vi "Update.vi"(8 "error in (no error)":errorcluster, 11 "Deck in":refnum<class "Deck.lvclass">) -> (0 "error out":errorcluster, 2 "Audio Block":dbl[][](array[numeric]), 3 "Deck out":refnum<class "Deck.lvclass">)   [LabVIEW 2019, in "Deck.lvclass"]
uses:
  Deck.lvclass
  Deck.lvclass/Deck.ctl
  State.ctl
  Libraries/Audio Processing/Adjust Sample Size.vi
  Libraries/Globals/Constants.vi
  <vilib>/gmath/NI_Gmath.lvlib
  Libraries/User Interface/User Interface.lvlib
  Libraries/Audio Processing/Audio Processing.lvlib
  Libraries/Messaging/Messaging.lvlib
  Libraries/Globals/Globals.lvlib
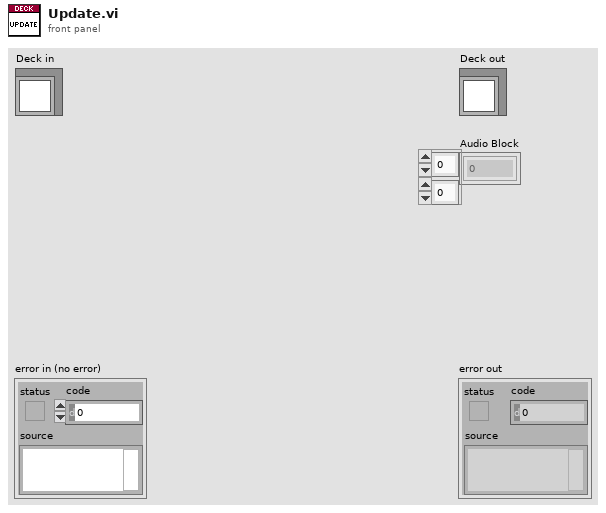
[diagram p1: front panel]
types:
  T1 = typedef "Deck.lvclass/State.ctl" = enum16{"No Track", "Loading", "Active", "Scratching", "Brake", "Backspin"}
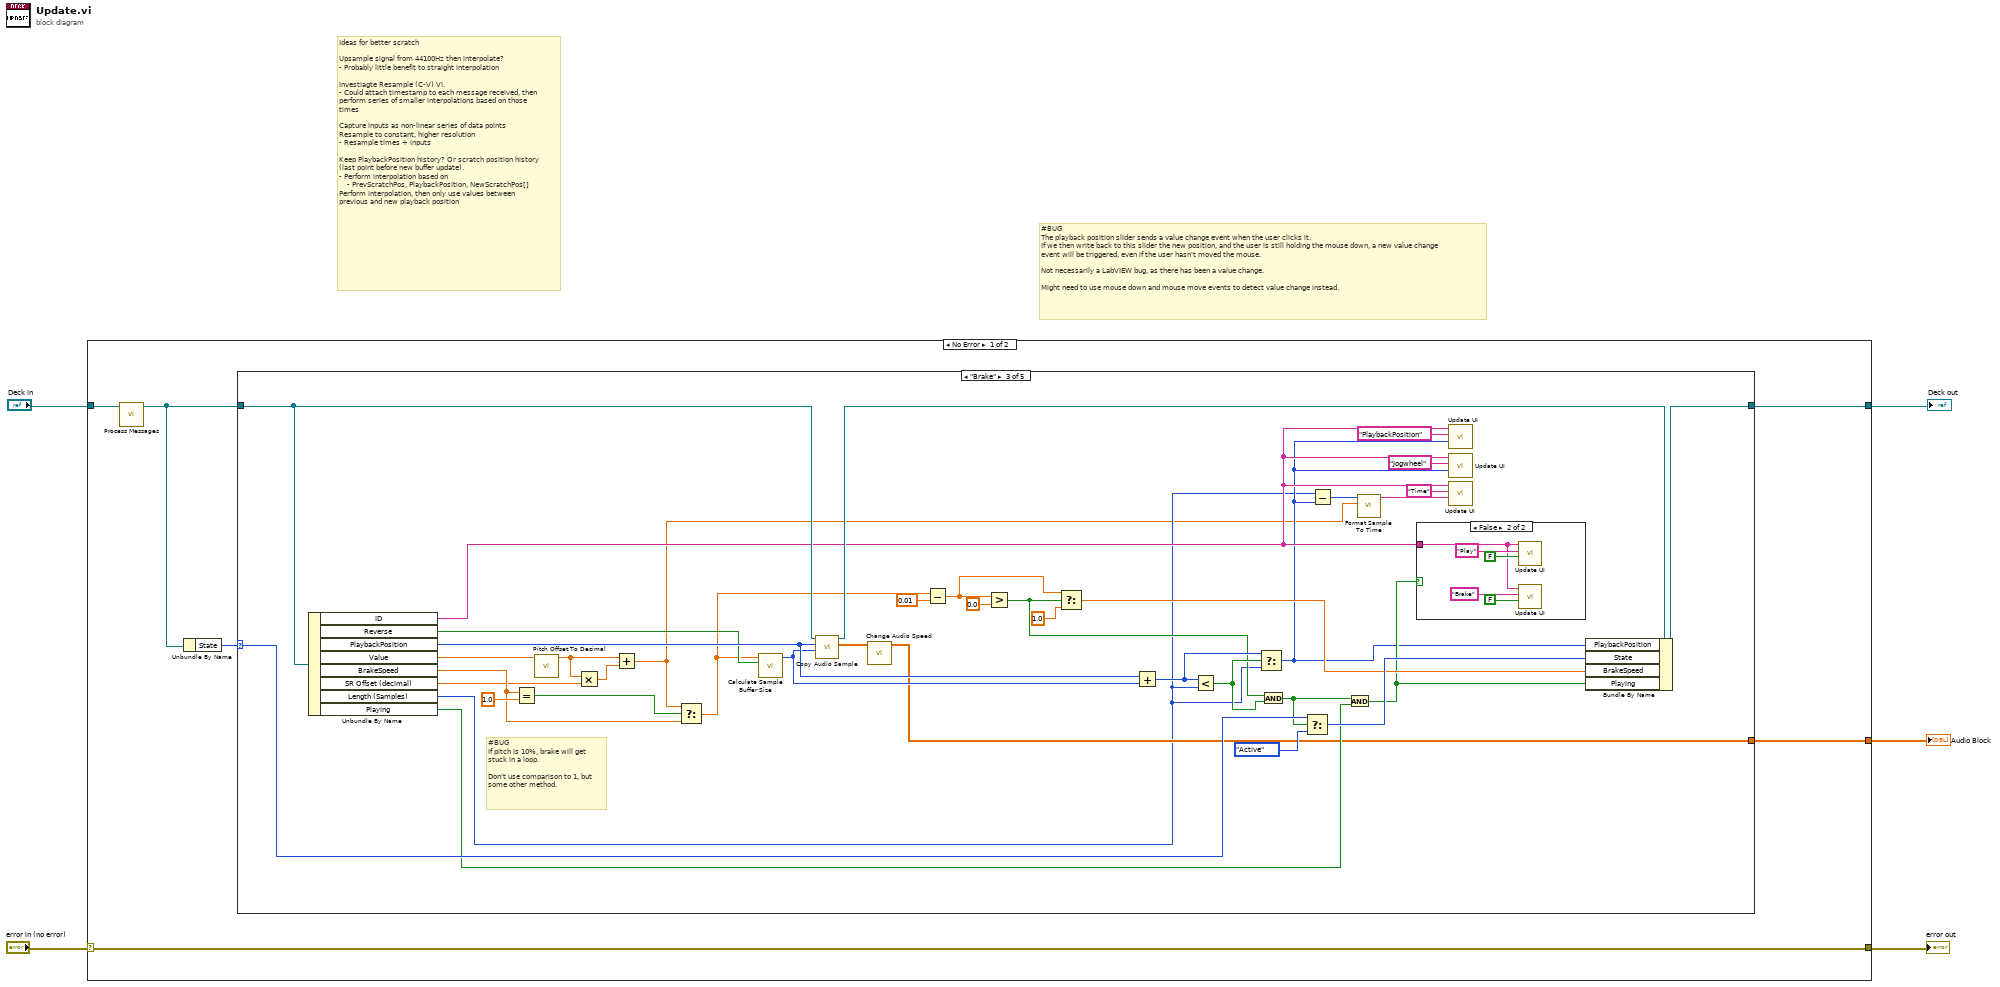
[diagram p0: block diagram]
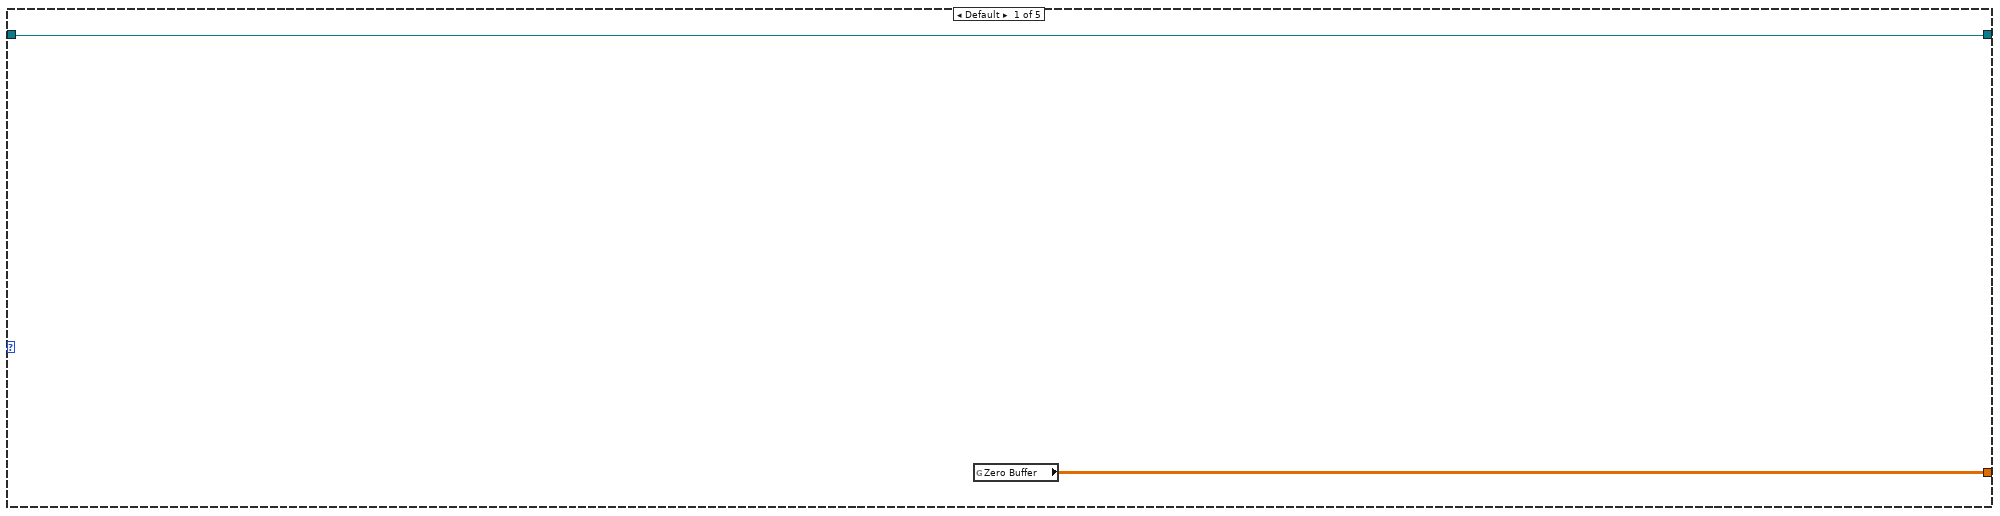
[diagram p2: hidden frame]
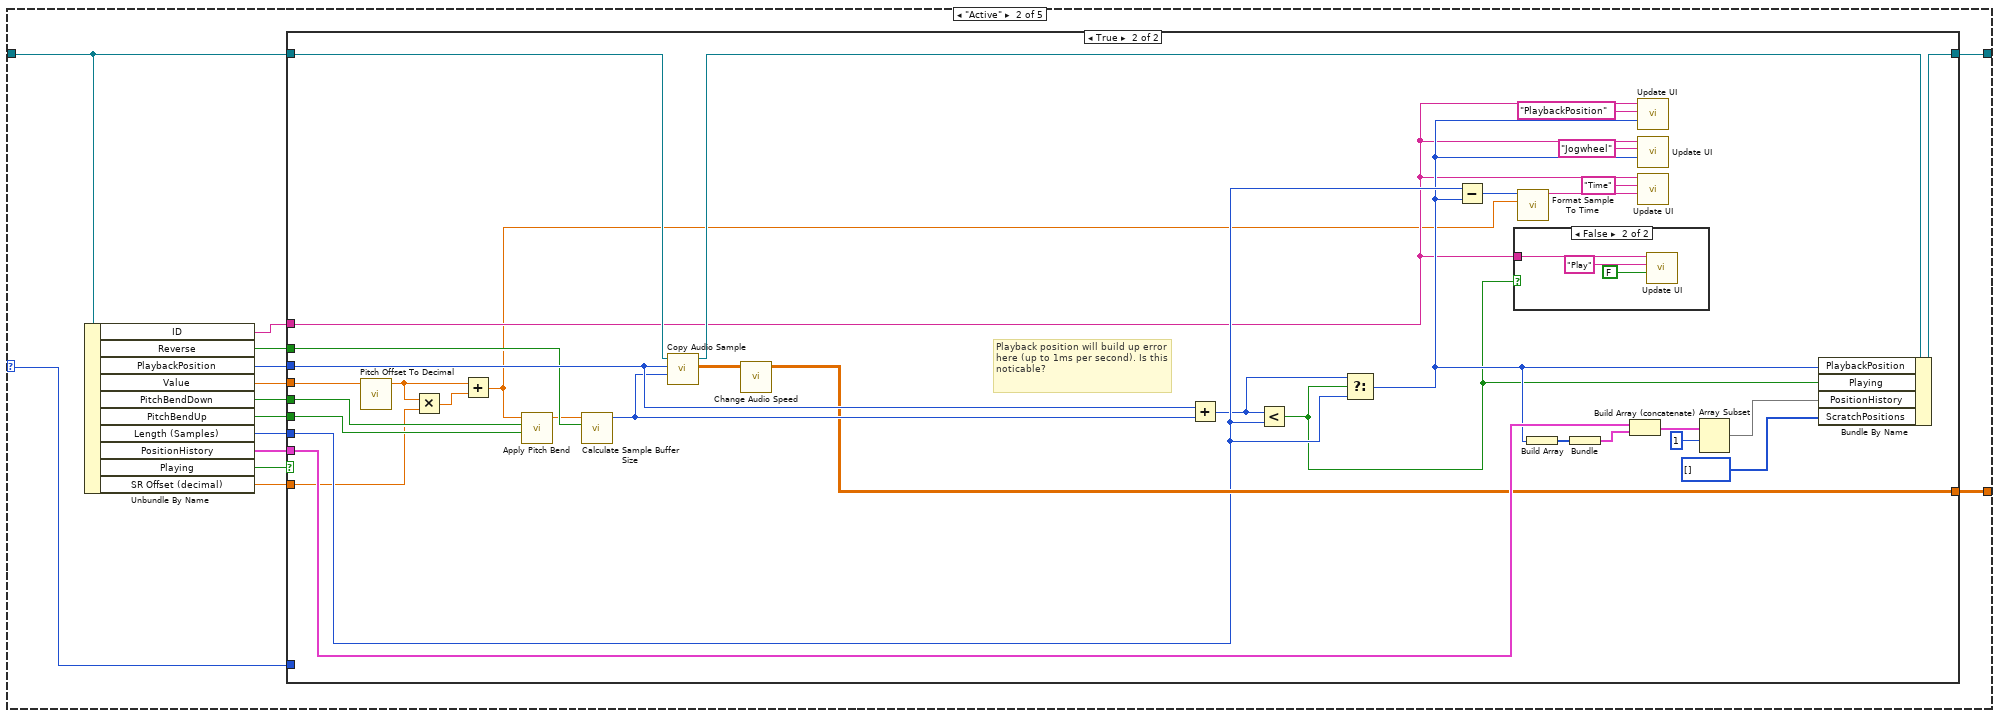
[diagram p3: hidden frame]
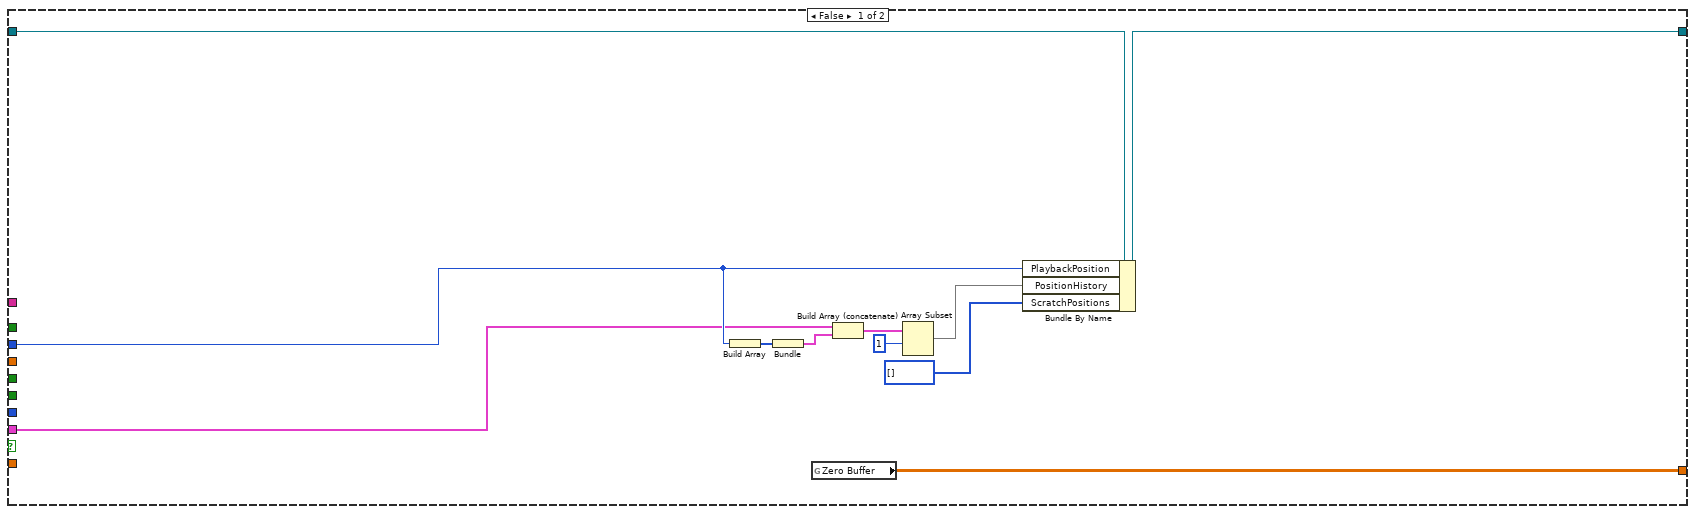
[diagram p4: hidden frame]
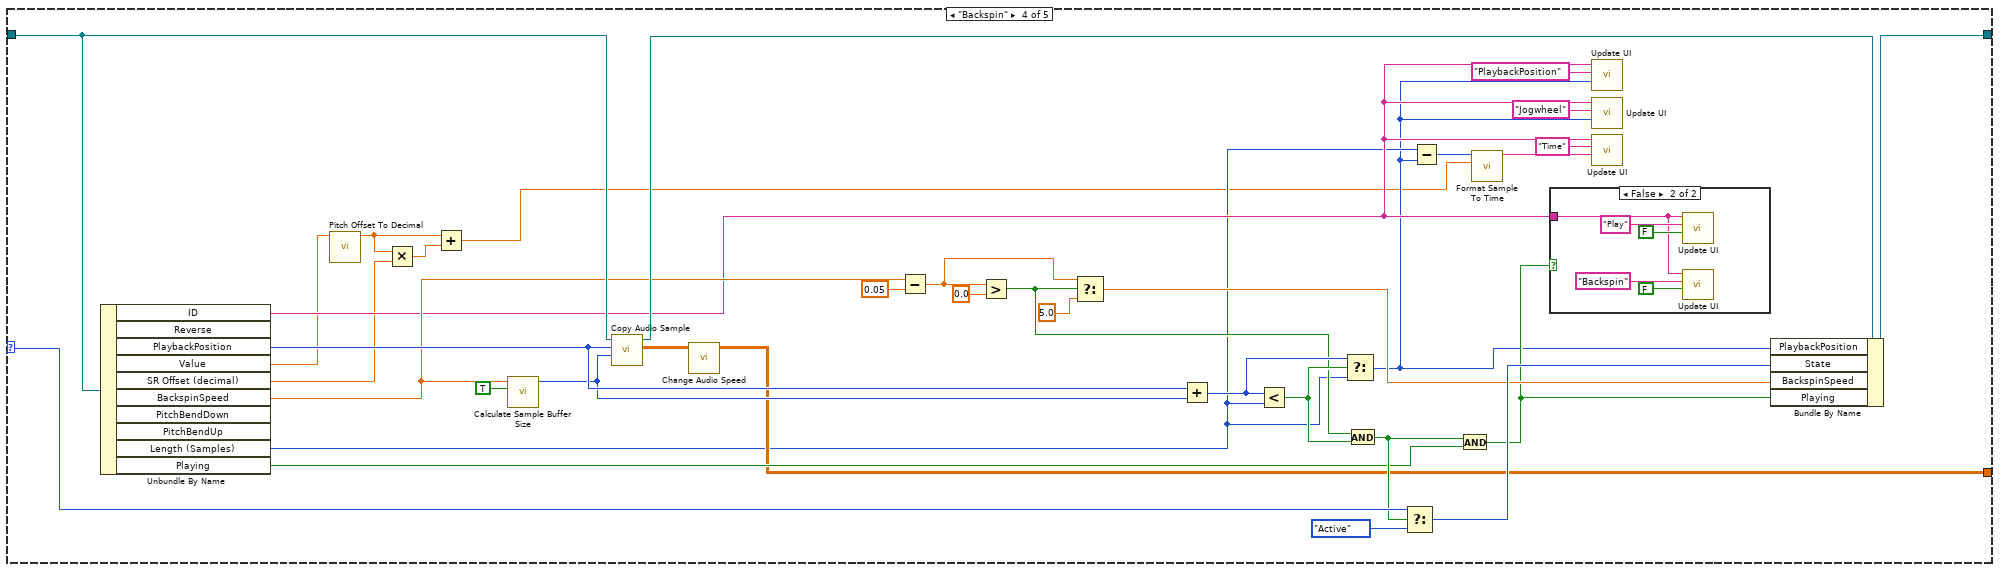
[diagram p7: hidden frame]
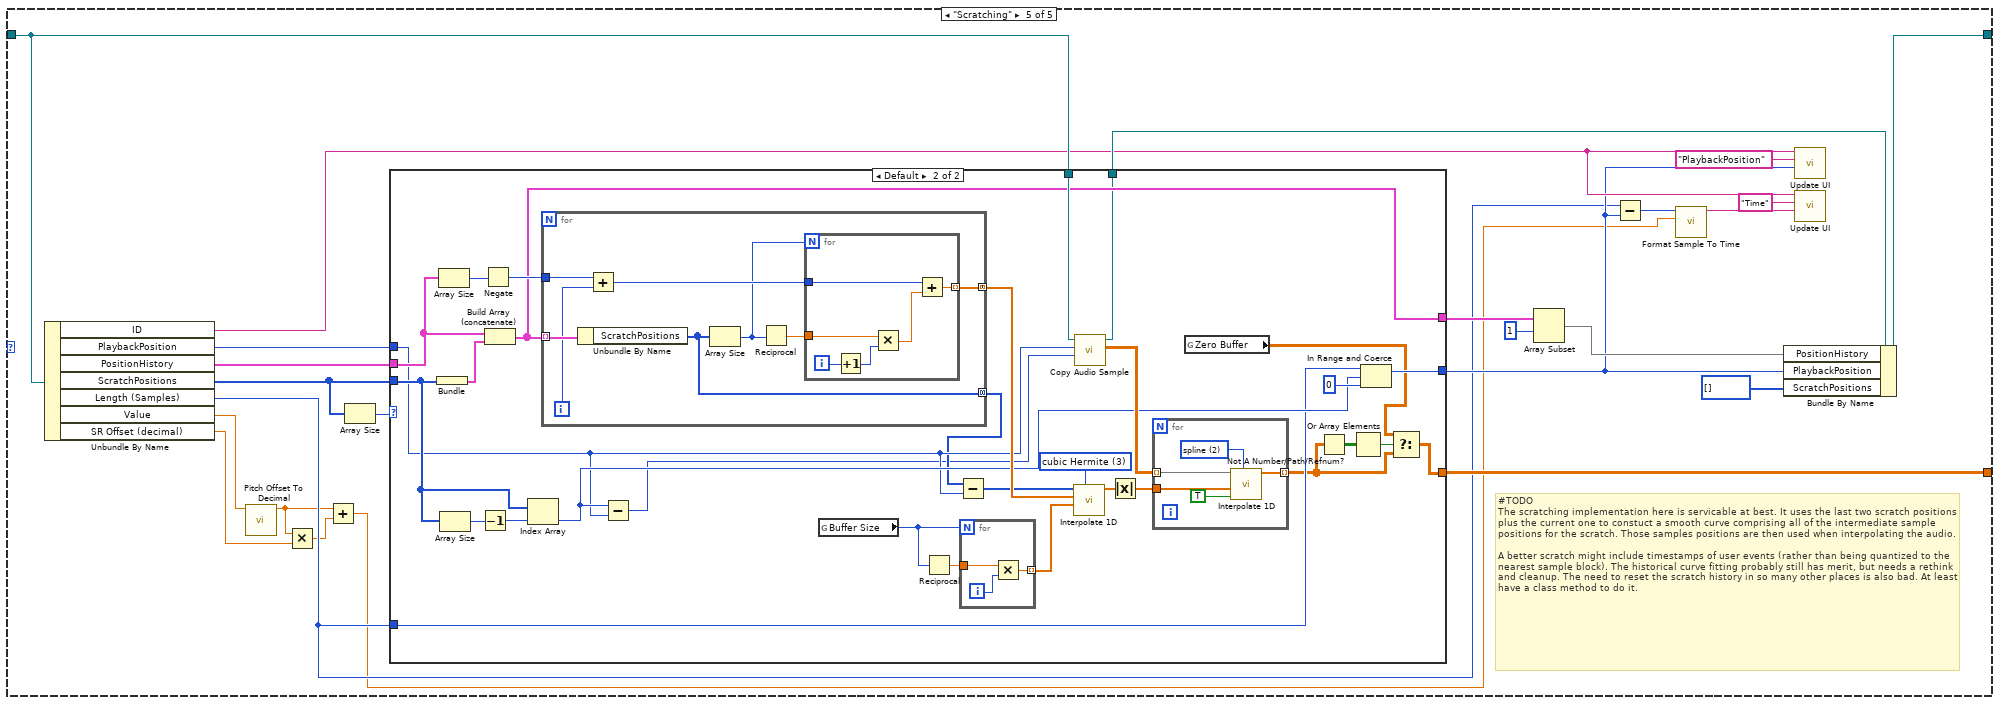
[diagram p9: hidden frame]
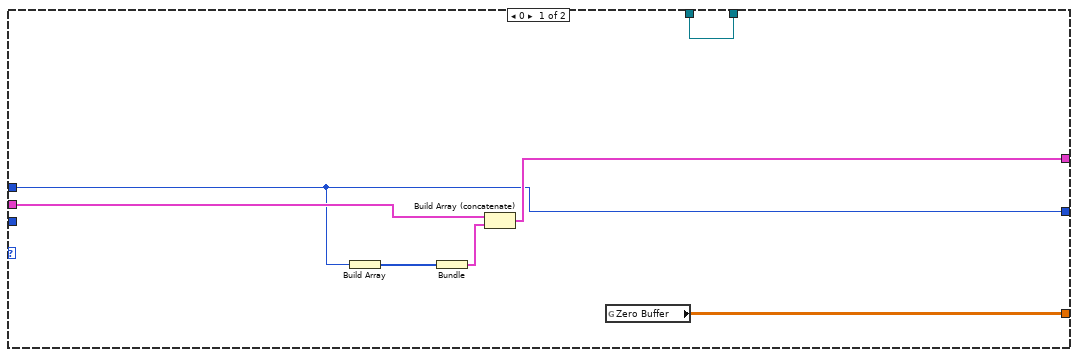
[diagram p10: hidden frame]
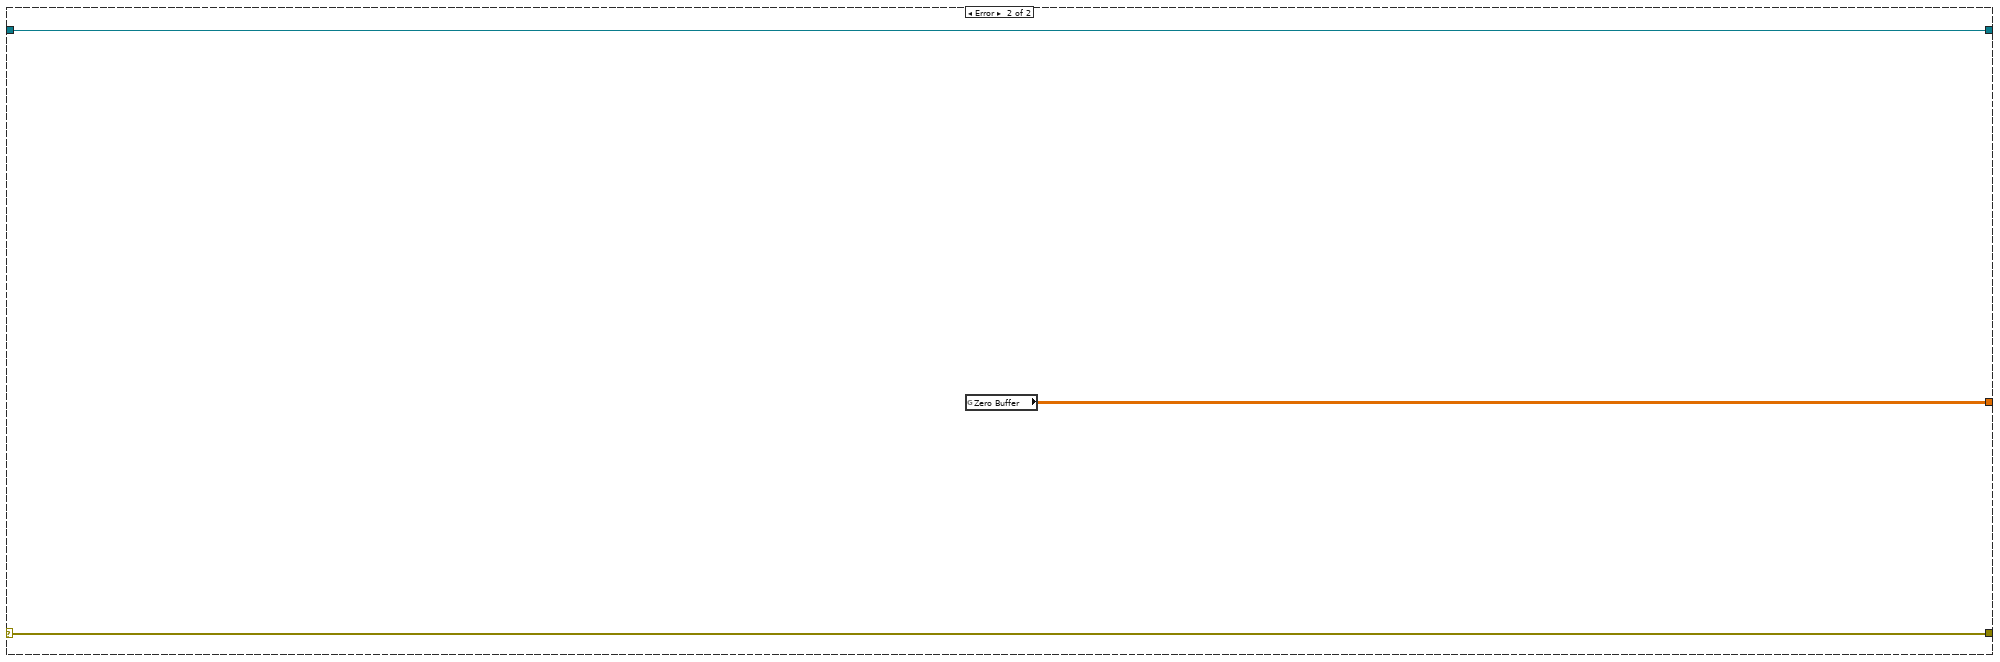
[diagram p11: hidden frame]
diagram:
  # "Ideas for better scratch\n\nUpsample signal from 44100Hz then interpolate?\n- Probably little benefit to straight interpolation\n\nInvestiagte Resample (C-V) VI.\n- Could attach timestamp to each message received, then perform series of smaller interpolations based on those times\n\nCapture inputs as non-linear series of data points\nResample to constant, higher resolution\n- Resample times + inputs\n\nKeep PlaybackPosition history? Or scratch position history (last point before new buffer update).\n- Perform interpolation based on\n    - PrevScratchPos, PlaybackPosition, NewScratchPos[]\nPerform interpolation, then only use values between previous and new playback position"
  # "#BUG\nThe playback position slider sends a value change event when the user clicks it.\nIf we then write back to this slider the new position, and the user is still holding the mouse down, a new value change event will be triggered, even if the user hasn't moved the mouse.\n\nNot necessarily a LabVIEW bug, as there has been a value change.\n\nMight need to use mouse down and mouse move events to detect value change instead."
  n1 = case shown="No Error" "error in (no error)" {
    selector: "error in (no error)" -> [w11 w246]
    tunnel: [w11 w246] -> w4
    tunnel: [w9 w245] -> w2
    tunnel: "Deck in" -> [w6 w245]
    tunnel: [w8 w244] -> w1
    frame No Error {
      n2 = call "Process Messages.vi"("Deck in"=w6) -> ("Deck out"=w7:refnum<class "Deck.lvclass">)  [unwired: 9 in, 1 out]
      n3 = Unbundle By Name(w7) -> ("State"=w10:T1)
      n4 = case shown="\"Brake\"" w10 {
        selector: w10 -> [_ w20 w108 w149 _]
        tunnel: [w13 w27 w113 w154 w183] -> w9
        tunnel: w7 -> [w13 w26 w111 w152 w181]
        tunnel: [w12 w24 w87 w133 w172] -> w8
        frame Default {
          n5 = global read "Constants.vi" "Zero Buffer"() -> (w12:dbl[][])
        }
        frame "Active" {
          n6 = Unbundle By Name(w26) -> ("ID"=w16:string, "Reverse"=w15:bool, "PlaybackPosition"=w25:i32, "Value"=w22:dbl, "PitchBendDown"=w23:bool, "PitchBendUp"=w21:bool, "Length (Samples)"=w18:i32, "PositionHistory"=w19:cluster{"Positions":i32[]}[], "Playing"=w17:bool, "SR Offset (decimal)"=w14:dbl)
          n7 = case shown="True" w17 {
            tunnel: [w31 w71] -> w27
            tunnel: w26 -> [w30 w69]
            tunnel: w25 -> [w29 w68]
            tunnel: [w38 w56] -> w24
            tunnel: w23 -> [_ w42]
            tunnel: w22 -> [_ w60]
            tunnel: w21 -> [_ w43]
            tunnel: w20 -> [_ _]
            tunnel: w19 -> [w28 w65]
            tunnel: w16 -> [_ w46]
            tunnel: w18 -> [_ w55]
            tunnel: w15 -> [_ w59]
            tunnel: w14 -> [_ w41]
            frame False {
              n8 = Build Array(w29) -> (w34:i32[])
              n9 = Bundle(w34) -> (w33:cluster{i32[]})  [unwired: 1 in]
              n10 = global read "Constants.vi" "Zero Buffer"() -> (w38:dbl[][])
              n11 = Build Array (concatenate)(w28, w33) -> (w37:cluster{"Positions":i32[]}[])
              n12 = Array Subset(array=w37, index=1) -> (w35:cluster{"Positions":i32[]}[])  [unwired: 1 in]
              n13 = Bundle By Name(cluster=w30, "PlaybackPosition"=w29, "PositionHistory"=w35, "ScratchPositions"=i32[] []) -> (w31:refnum<class "Deck.lvclass">)
            }
            frame True {
              # "Playback position will build up error here (up to 1ms per second). Is this noticable?"
              n14 = call "Pitch Offset To Decimal.vi"("Pitch Offset (%)"=w60) -> ("Pitch (decimal)"=w40:dbl)  [unwired: 10 in]
              n15 = Multiply(x=w40, y=w41) -> (x*y=w39:dbl)
              n16 = Add(x=w40, y=w39) -> (x+y=w45:dbl)
              n17 = call "Apply Pitch Bend.vi"("Pitch Bend Up (F)"=w43, "Pitch Bend Down (F)"=w42, "Pitch (decimal) In"=w45) -> ("Pitch (decimal) Out"=w44:dbl)  [unwired: 8 in]
              n18 = call "Calculate Sample Buffer Size.vi"("Reverse (F)"=w59, "Speed Multiplier"=w44) -> ("Sample Size"=w58:i32)  [unwired: 9 in]
              n19 = call "Copy Audio Sample.vi"("Length"=w58, "Offset"=w68, "Deck in"=w69) -> ("Audio Block"=w57:dbl[][], "Deck out"=w70:refnum<class "Deck.lvclass">)  [unwired: 6 in, 1 out]
              n20 = call "Change Audio Speed.vi"("Audio Block"=w57) -> ("Interpolated Audio"=w56:dbl[][])  [unwired: 10 in]
              n21 = Add(x=w68, y=w58) -> (x+y=w54:i32)
              n22 = Less?(x=w54, y=w55) -> (x < y?=w47:bool)
              n23 = Select(t=w54, s=w47, f=w55) -> (s? t:f=w50:i32)
              n24 = Subtract(x=w55, y=w50) -> (x-y=w53:i32)
              n25 = case shown="False" w47 {
                tunnel: w46 -> [_ w72]
                frame True {
                }
                frame False {
                  n26 = call "Update UI.vi"("Data"=FALSE, "Target"="Play" ("format string"), "ID"=w72) -> ()  [unwired: 8 in, 1 out]
                }
              }
              n27 = call "Format Sample To Time.vi"("Pitch (decimal) (1)"=w45, "Samples"=w53) -> ("Formatted Time"=w49:string)  [unwired: 9 in]
              n28 = Build Array(w50) -> (w63:i32[])
              n29 = Bundle(w63) -> (w62:cluster{i32[]})  [unwired: 1 in]
              n30 = Build Array (concatenate)(w65, w62) -> (w67:cluster{"Positions":i32[]}[])
              n31 = call "Update UI.vi"("Data"=w50, "Target"="PlaybackPosition" ("format string"), "ID"=w46) -> ()  [unwired: 8 in, 1 out]
              n32 = call "Update UI.vi"("Data"=w50, "Target"="Jogwheel" ("format string"), "ID"=w46) -> ()  [unwired: 8 in, 1 out]
              n33 = call "Update UI.vi"("Data"=w49, "Target"="Time" ("format string"), "ID"=w46) -> ()  [unwired: 8 in, 1 out]
              n34 = Array Subset(array=w67, index=1) -> (w64:cluster{"Positions":i32[]}[])  [unwired: 1 in]
              n35 = Bundle By Name(cluster=w70, "PlaybackPosition"=w50, "Playing"=w47, "PositionHistory"=w64, "ScratchPositions"=i32[] []) -> (w71:refnum<class "Deck.lvclass">)
            }
          }
        }
        frame "Brake" {
          # "#BUG\nIf pitch is 10%, brake will get stuck in a loop.\n\nDon't use comparison to 1, but some other method."
          n36 = Unbundle By Name(w111) -> ("ID"=w81:string, "Reverse"=w90:bool, "PlaybackPosition"=w110:i32, "Value"=w92:dbl, "BrakeSpeed"=w96:dbl, "SR Offset (decimal)"=w76:dbl, "Length (Samples)"=w79:i32, "Playing"=w94:bool)
          n37 = Equal?(x=w96, y=1.0) -> (x = y?=w97:bool)
          n38 = call "Pitch Offset To Decimal.vi"("Pitch Offset (%)"=w92) -> ("Pitch (decimal)"=w77:dbl)  [unwired: 10 in]
          n39 = Multiply(x=w77, y=w76) -> (x*y=w78:dbl)
          n40 = Add(x=w77, y=w78) -> (x+y=w75:dbl)
          n41 = Select(t=w75, s=w97, f=w96) -> (s? t:f=w89:dbl)
          n42 = call "Calculate Sample Buffer Size.vi"("Reverse (F)"=w90, "Speed Multiplier"=w89) -> ("Sample Size"=w88:i32)  [unwired: 9 in]
          n43 = call "Copy Audio Sample.vi"("Length"=w88, "Offset"=w110, "Deck in"=w111) -> ("Audio Block"=w91:dbl[][], "Deck out"=w112:refnum<class "Deck.lvclass">)  [unwired: 6 in, 1 out]
          n44 = call "Change Audio Speed.vi"("Audio Block"=w91) -> ("Interpolated Audio"=w87:dbl[][])  [unwired: 10 in]
          n45 = Subtract(x=w89, y=0.01) -> (x-y=w99:dbl)
          n46 = Greater?(x=w99, y=0.0) -> (0:w102:bool)
          n47 = Select(t=w99, s=w102, f=1.0 ("t")) -> (s? t:f=w101:dbl)
          n48 = Add(x=w110, y=w88) -> (x+y=w109:i32)
          n49 = Less?(x=w109, y=w79) -> (x < y?=w103:bool)
          n50 = Select(t=w109, s=w103, f=w79) -> (s? t:f=w80:i32)
          n51 = And(x=w102, y=w103) -> (x .and. y?=w95:bool)
          n52 = Select(t=w108, s=w95, f=State."Active") -> (s? t:f=w107:T1)
          n53 = Subtract(x=w79, y=w80) -> (x-y=w86:i32)
          n54 = And(x=w95, y=w94) -> (x .and. y?=w93:bool)
          n55 = call "Format Sample To Time.vi"("Pitch (decimal) (1)"=w75, "Samples"=w86) -> ("Formatted Time"=w83:string)  [unwired: 9 in]
          n56 = case shown="False" w93 {
            tunnel: w81 -> [_ w114]
            frame True {
            }
            frame False {
              n57 = call "Update UI.vi"("Data"=FALSE, "Target"="Play" ("format string"), "ID"=w114) -> ()  [unwired: 8 in, 1 out]
              n58 = call "Update UI.vi"("Data"=FALSE, "Target"="Brake" ("format string"), "ID"=w114) -> ()  [unwired: 8 in, 1 out]
            }
          }
          n59 = call "Update UI.vi"("Data"=w80, "Target"="PlaybackPosition" ("format string"), "ID"=w81) -> ()  [unwired: 8 in, 1 out]
          n60 = call "Update UI.vi"("Data"=w80, "Target"="Jogwheel" ("format string"), "ID"=w81) -> ()  [unwired: 8 in, 1 out]
          n61 = call "Update UI.vi"("Data"=w83, "Target"="Time" ("format string"), "ID"=w81) -> ()  [unwired: 8 in, 1 out]
          n62 = Bundle By Name(cluster=w112, "PlaybackPosition"=w80, "State"=w107, "BrakeSpeed"=w101, "Playing"=w93) -> (w113:refnum<class "Deck.lvclass">)
        }
        frame "Backspin" {
          n63 = Unbundle By Name(w152) -> ("ID"=w127:string, "PlaybackPosition"=w151:i32, "Value"=w123:dbl, "SR Offset (decimal)"=w121:dbl, "BackspinSpeed"=w137:dbl, "Length (Samples)"=w125:i32, "Playing"=w138:bool)  [unwired: 3 out]
          n64 = call "Pitch Offset To Decimal.vi"("Pitch Offset (%)"=w123) -> ("Pitch (decimal)"=w119:dbl)  [unwired: 10 in]
          n65 = Multiply(x=w119, y=w121) -> (x*y=w122:dbl)
          n66 = Add(x=w119, y=w122) -> (x+y=w120:dbl)
          n67 = call "Calculate Sample Buffer Size.vi"("Reverse (F)"=TRUE, "Speed Multiplier"=w137) -> ("Sample Size"=w135:i32)  [unwired: 9 in]
          n68 = call "Copy Audio Sample.vi"("Length"=w135, "Offset"=w151, "Deck in"=w152) -> ("Audio Block"=w134:dbl[][], "Deck out"=w153:refnum<class "Deck.lvclass">)  [unwired: 6 in, 1 out]
          n69 = call "Change Audio Speed.vi"("Audio Block"=w134) -> ("Interpolated Audio"=w133:dbl[][])  [unwired: 10 in]
          n70 = Subtract(x=w137, y=0.05) -> (x-y=w140:dbl)
          n71 = Greater?(x=w140, y=0.0) -> (0:w143:bool)
          n72 = Select(t=w140, s=w143, f=5.0 ("t")) -> (s? t:f=w142:dbl)
          n73 = Add(x=w151, y=w135) -> (x+y=w150:i32)
          n74 = Less?(x=w150, y=w125) -> (x < y?=w144:bool)
          n75 = Select(t=w150, s=w144, f=w125) -> (s? t:f=w124:i32)
          n76 = And(x=w143, y=w144) -> (x .and. y?=w139:bool)
          n77 = Select(t=w149, s=w139, f=State."Active") -> (s? t:f=w148:T1)
          n78 = Subtract(x=w125, y=w124) -> (x-y=w132:i32)
          n79 = And(x=w139, y=w138) -> (x .and. y?=w126:bool)
          n80 = call "Format Sample To Time.vi"("Pitch (decimal) (1)"=w120, "Samples"=w132) -> ("Formatted Time"=w129:string)  [unwired: 9 in]
          n81 = case shown="False" w126 {
            tunnel: w127 -> [_ w155]
            frame True {
            }
            frame False {
              n82 = call "Update UI.vi"("Data"=FALSE, "Target"="Play" ("format string"), "ID"=w155) -> ()  [unwired: 8 in, 1 out]
              n83 = call "Update UI.vi"("Data"=FALSE, "Target"="Backspin" ("format string"), "ID"=w155) -> ()  [unwired: 8 in, 1 out]
            }
          }
          n84 = call "Update UI.vi"("Data"=w124, "Target"="PlaybackPosition" ("format string"), "ID"=w127) -> ()  [unwired: 8 in, 1 out]
          n85 = call "Update UI.vi"("Data"=w124, "Target"="Jogwheel" ("format string"), "ID"=w127) -> ()  [unwired: 8 in, 1 out]
          n86 = call "Update UI.vi"("Data"=w129, "Target"="Time" ("format string"), "ID"=w127) -> ()  [unwired: 8 in, 1 out]
          n87 = Bundle By Name(cluster=w153, "PlaybackPosition"=w124, "State"=w148, "BackspinSpeed"=w142, "Playing"=w126) -> (w154:refnum<class "Deck.lvclass">)
        }
        frame "Scratching" {
          # "#TODO\nThe scratching implementation here is servicable at best. It uses the last two scratch positions plus the current one to constuct a smooth curve comprising all of the intermediate sample positions for the scratch. Those samples positions are then used when interpolating the audio.\n\nA better scratch might include timestamps of user events (rather than being quantized to the nearest sample block). The historical curve fitting probably still has merit, but needs a rethink and cleanup. The need to reset the scratch history in so many other places is also bad. At least have a class method to do it."
          n88 = Unbundle By Name(w181) -> ("ID"=w167:string, "PlaybackPosition"=w180:i32, "PositionHistory"=w179:cluster{"Positions":i32[]}[], "ScratchPositions"=w177:i32[], "Length (Samples)"=w165:i32, "Value"=w164:dbl, "SR Offset (decimal)"=w162:dbl)
          n89 = call "Pitch Offset To Decimal.vi"("Pitch Offset (%)"=w164) -> ("Pitch (decimal)"=w160:dbl)  [unwired: 10 in]
          n90 = Multiply(x=w160, y=w162) -> (x*y=w163:dbl)
          n91 = Add(x=w160, y=w163) -> (x+y=w161:dbl)
          n92 = Array Size(array=w177) -> (size(s)=w178:i32)
          n93 = case shown="Default" w178 {
            tunnel: [w186 w220] -> w166
            tunnel: [w190 w197] -> w182
            tunnel: w181 -> [w190 w221]
            tunnel: w180 -> [w186 w203]
            tunnel: [w184 w193] -> w172
            tunnel: w165 -> [_ w199]
            tunnel: w179 -> [w187 w213]
            tunnel: [w188 w204] -> w176
            tunnel: w177 -> [_ w209]
            frame 0 {
              n94 = Build Array(w186) -> (w185:i32[])
              n95 = Bundle(w185) -> (w189:cluster{i32[]})  [unwired: 1 in]
              n96 = Build Array (concatenate)(w187, w189) -> (w188:cluster{"Positions":i32[]}[])
              n97 = global read "Constants.vi" "Zero Buffer"() -> (w184:dbl[][])
            }
            frame Default {
              w215 = 3 items=["nearest", "linear", "spline", "cubic Hermite", "Lagrange"] ("method")
              n98 = Bundle("ScratchPositions"=w209) -> (w214:cluster{"ScratchPositions":i32[]})  [unwired: 1 in]
              n99 = Array Size(array=w213) -> (size(s)=w217:i32)
              n100 = Array Size(array=w209) -> (size(s)=w211:i32)
              n101 = Decrement(x=w211) -> (x-1=w210:i32)
              n102 = Negate(x=w217) -> (-x=w216:i32)
              n103 = Build Array (concatenate)(w213, w214) -> (w204:cluster{"ScratchPositions":i32[]}[])
              n104 = Index Array(array=w209, index=w210) -> (element=w205:i32)
              n105 = for {
                tunnel: w204 -> [w232] mode=indexing
                tunnel: w216 -> [w226]
                tunnel: [w230] -> w212 mode=concatenating
                tunnel: [w229] -> w201 mode=concatenating
                i -> [w228]
                n106 = Unbundle By Name(w232) -> ("ScratchPositions"=w229:i32[])
                n107 = Add(x=w226, y=w228) -> (x+y=w227:i32)
                n108 = Array Size(array=w229) -> (size(s)=w225:i32)
                n109 = Reciprocal(x=w225) -> (1/x=w231:dbl)
                n110 = for {
                  N: w225 -> [_]
                  tunnel: w231 -> [w235]
                  tunnel: w227 -> [w238]
                  tunnel: [w234] -> w230 mode=indexing
                  i -> [w237]
                  n111 = Increment(x=w237) -> (x+1=w233:i32)
                  n112 = Multiply(x=w235, y=w233) -> (x*y=w236:dbl)
                  n113 = Add(x=w238, y=w236) -> (x+y=w234:dbl)
                }
              }
              n114 = Subtract(x=w205, y=w203) -> (x-y=w198:i32)
              n115 = global read "Constants.vi" "Buffer Size"() -> (w192:i32)
              n116 = Reciprocal(x=w192) -> (1/x=w208:dbl)
              n117 = Subtract(x=w201, y=w203) -> (x-y=w202:i32[])
              n118 = for {
                N: w192 -> [_]
                tunnel: w208 -> [w223]
                tunnel: [w222] -> w207 mode=indexing
                i -> [w224]
                n119 = Multiply(x=w223, y=w224) -> (x*y=w222:dbl)
              }
              n120 = call <vilib>:"Interpolate 1D.vi"("method"=w215, "xi"=w207, "X"=w212, "Y"=w202) -> ("yi"=w206:dbl[])  [unwired: 5 in, 2 out]
              n121 = call "Copy Audio Sample.vi"("Length"=w198, "Offset"=w203, "Deck in"=w221) -> ("Audio Block"=w219:dbl[][], "Deck out"=w197:refnum<class "Deck.lvclass">)  [unwired: 6 in, 1 out]
              n122 = Absolute Value(x=w206) -> (abs(x)=w200:dbl[])
              n123 = for {
                tunnel: w219 -> [w239] mode=indexing
                tunnel: w200 -> [w240]
                tunnel: [w241] -> w194 mode=indexing
                w242 = 2 items=["nearest", "linear", "spline", "cubic Hermite", "Lagrange"] ("method")
                n124 = call <vilib>:"Interpolate 1D.vi"("method"=w242, "X is monotonic"=TRUE, "xi"=w240, "Y"=w239) -> ("yi"=w241:dbl[])  [unwired: 5 in, 2 out]
              }
              n125 = global read "Constants.vi" "Zero Buffer"() -> (w191:dbl[][])
              n126 = Not A Number/Path/Refnum?(number/path/refnum=w194) -> (NaN/Path/Refnum?=w196:bool[][])
              n127 = Or Array Elements(Boolean array=w196) -> (logical OR=w195:bool)
              n128 = In Range and Coerce(upper limit=w199, x=w205, lower limit=0) -> (coerced(x)=w220:i32)  [unwired: 1 out]
              n129 = Select(t=w191, s=w195, f=w194) -> (s? t:f=w193:dbl[][])
            }
          }
          n130 = Array Subset(array=w176, index=1) -> (w174:cluster{"ScratchPositions":i32[]}[])  [unwired: 1 in]
          n131 = Subtract(x=w165, y=w166) -> (x-y=w171:i32)
          n132 = call "Format Sample To Time.vi"("Pitch (decimal) (1)"=w161, "Samples"=w171) -> ("Formatted Time"=w169:string)  [unwired: 9 in]
          n133 = Bundle By Name(cluster=w182, "PositionHistory"=w174, "PlaybackPosition"=w166, "ScratchPositions"=i32[] []) -> (w183:refnum<class "Deck.lvclass">)
          n134 = call "Update UI.vi"("Data"=w166, "Target"="PlaybackPosition" ("format string"), "ID"=w167) -> ()  [unwired: 8 in, 1 out]
          n135 = call "Update UI.vi"("Data"=w169, "Target"="Time" ("format string"), "ID"=w167) -> ()  [unwired: 8 in, 1 out]
        }
      }
    }
    frame Error {
      n136 = global read "Constants.vi" "Zero Buffer"() -> (w244:dbl[][])
    }
  }
  "error out" <- w4
  "Deck out" <- w2
  "Audio Block" <- w1
